vi "DEMO1.vi"() -> ()   [LabVIEW 2018]
uses:
  <vilib>/Utility/miscctls.llb/LVPositionTypeDef.ctl
  RandomMoveBool.lvclass
  RandomMoveBool.lvclass/RandomMoveBool.ctl
panel:
  out "数值":i32
  in  "Color":u32(colorbox)=6618880
  in  "Stop":bool
  in  "Remove":bool
  in  "Add":bool
  out "10 9":bool caption="布尔6"
  out "5 9":bool caption="布尔5"
  out "3 9":bool caption="布尔4"
  out "4 9":bool caption="布尔5"
  out "6 9":bool caption="布尔3"
  out "9 9":bool caption="布尔4"
  out "7 9":bool caption="布尔6"
  out "2 9":bool caption="布尔5"
  out "1 9":bool caption="布尔4"
  out "8 9":bool caption="布尔7"
  out "10 10":bool caption="布尔6"
  out "5 10":bool caption="布尔5"
  out "3 10":bool caption="布尔4"
  out "4 10":bool caption="布尔5"
  out "6 10":bool caption="布尔3"
  out "9 10":bool caption="布尔4"
  out "7 10":bool caption="布尔6"
  out "2 10":bool caption="布尔5"
  out "1 10":bool caption="布尔4"
  out "8 10":bool caption="布尔7"
  out "10 5":bool caption="布尔6"
  out "5 5":bool caption="布尔5"
  out "3 5":bool caption="布尔4"
  out "4 5":bool caption="布尔5"
  out "6 5":bool caption="布尔3"
  out "9 5":bool caption="布尔4"
  out "7 5":bool caption="布尔6"
  out "2 5":bool caption="布尔5"
  out "1 5":bool caption="布尔4"
  out "8 5":bool caption="布尔7"
  out "10 6":bool caption="布尔6"
  out "5 6":bool caption="布尔5"
  out "3 6":bool caption="布尔4"
  out "4 6":bool caption="布尔5"
  out "6 6":bool caption="布尔3"
  out "9 6":bool caption="布尔4"
  out "7 6":bool caption="布尔6"
  out "2 6":bool caption="布尔5"
  out "1 6":bool caption="布尔4"
  out "8 6":bool caption="布尔7"
  out "10 7":bool caption="布尔6"
  out "5 7":bool caption="布尔5"
  out "3 7":bool caption="布尔4"
  out "4 7":bool caption="布尔5"
  out "6 7":bool caption="布尔3"
  out "9 7":bool caption="布尔4"
  out "7 7":bool caption="布尔6"
  out "2 7":bool caption="布尔5"
  out "1 7":bool caption="布尔4"
  out "8 7":bool caption="布尔7"
  out "10 8":bool caption="布尔6"
  out "5 8":bool caption="布尔5"
  out "3 8":bool caption="布尔4"
  out "4 8":bool caption="布尔5"
  out "6 8":bool caption="布尔3"
  out "9 8":bool caption="布尔4"
  out "7 8":bool caption="布尔6"
  out "2 8":bool caption="布尔5"
  out "1 8":bool caption="布尔4"
  out "8 8":bool caption="布尔7"
  out "10 3":bool caption="布尔6"
  out "5 3":bool caption="布尔5"
  out "3 3":bool caption="布尔4"
  out "4 3":bool caption="布尔5"
  out "6 3":bool caption="布尔3"
  out "9 3":bool caption="布尔4"
  out "7 3":bool caption="布尔6"
  out "2 3":bool caption="布尔5"
  out "1 3":bool caption="布尔4"
  out "8 3":bool caption="布尔7"
  out "10 4":bool caption="布尔6"
  out "5 4":bool caption="布尔5"
  out "3 4":bool caption="布尔4"
  out "4 4":bool caption="布尔5"
  out "6 4":bool caption="布尔3"
  out "9 4":bool caption="布尔4"
  out "7 4":bool caption="布尔6"
  out "2 4":bool caption="布尔5"
  out "1 4":bool caption="布尔4"
  out "8 4":bool caption="布尔7"
  out "10 2":bool caption="布尔6"
  out "5 2":bool caption="布尔5"
  out "3 2":bool caption="布尔4"
  out "4 2":bool caption="布尔5"
  out "6 2":bool caption="布尔3"
  out "9 2":bool caption="布尔4"
  out "7 2":bool caption="布尔6"
  out "2 2":bool caption="布尔5"
  out "1 2":bool caption="布尔4"
  out "8 2":bool caption="布尔7"
  out "10":bool caption="布尔6"
  out "5":bool caption="布尔5"
  out "3":bool caption="布尔4"
  out "4":bool caption="布尔5"
  out "6":bool caption="布尔3"
  out "9":bool caption="布尔4"
  out "7":bool caption="布尔6"
  out "2":bool caption="布尔5"
  out "1":bool caption="布尔4"
  out "8":bool caption="布尔7"
  out "数组":T1[](array[typedef])
  in  "frequency2":dbl=3.0 format="%#_13g"
  in  "frequency1":dbl=3.0 format="%#_13g"
  in  "?":enum16{"Random", "Sine", "Other"}(ring)
  in  "limit":dbl=150.0 format="%#_13g"
  in  "等待时间（毫秒）":u32 step=20
  in  "ChangeColor":bool
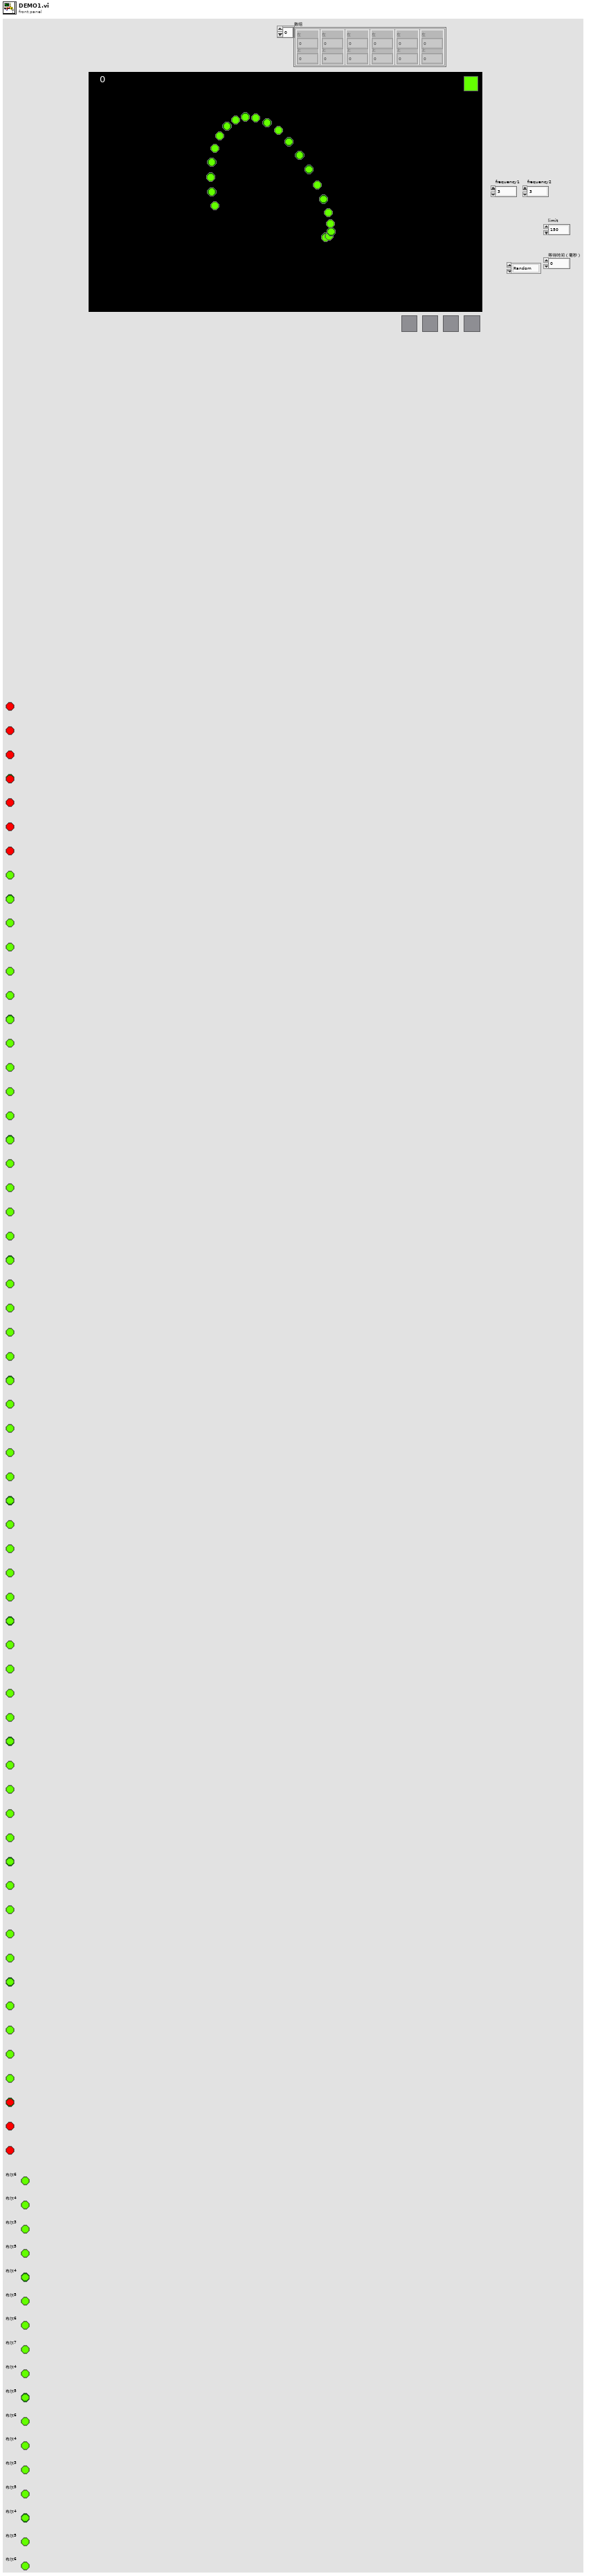
[diagram p1: front panel]
types:
  T1 = typedef "LVPositionTypeDef.ctl" = cluster{"Left":i32, "Top":i32}
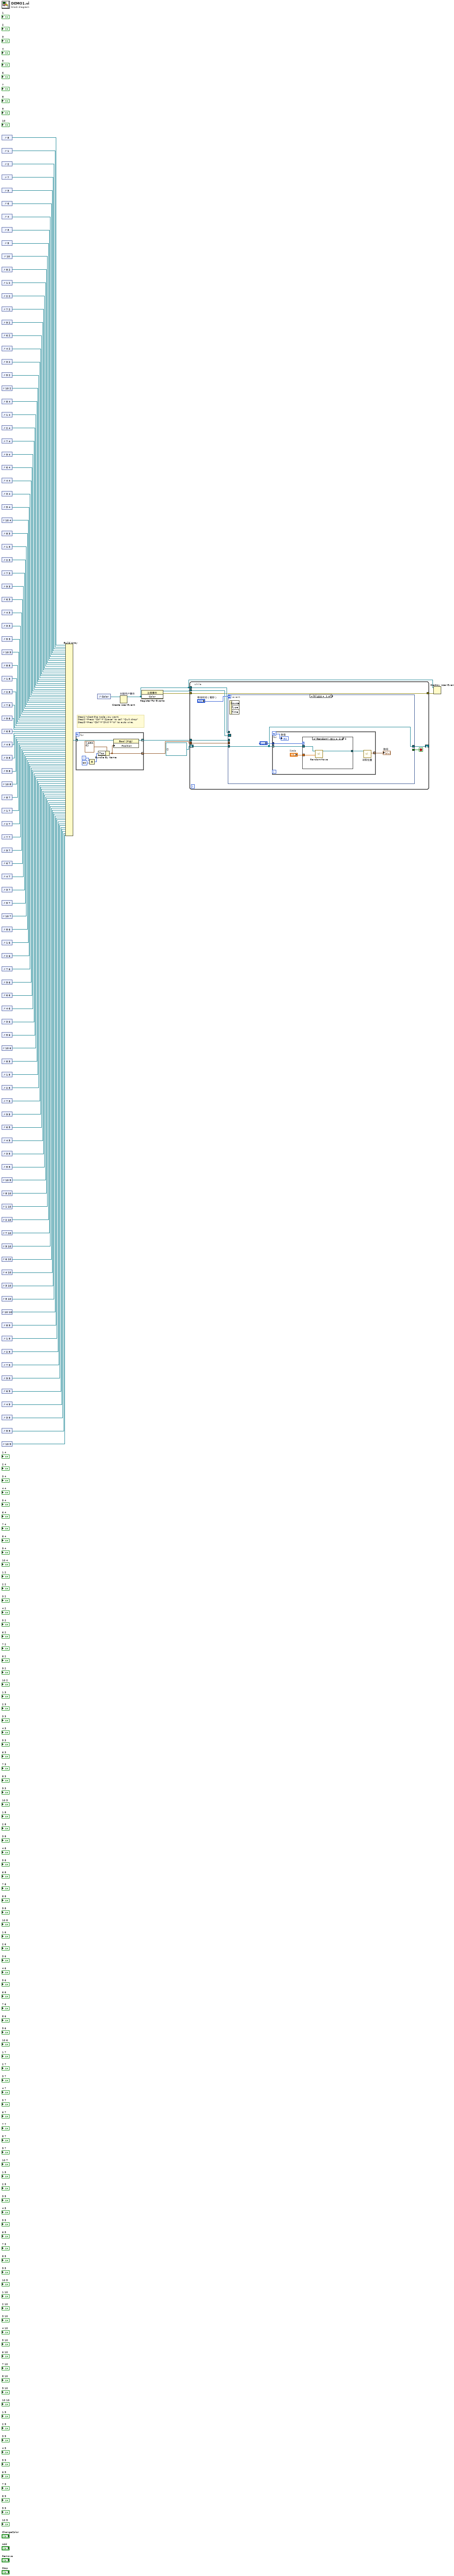
[diagram p0: block diagram]
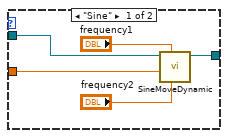
[diagram p2: hidden frame]
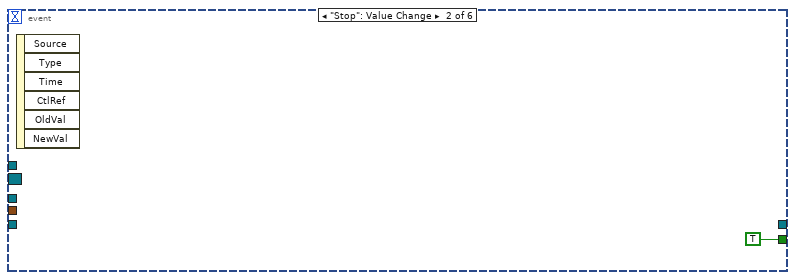
[diagram p3: hidden frame]
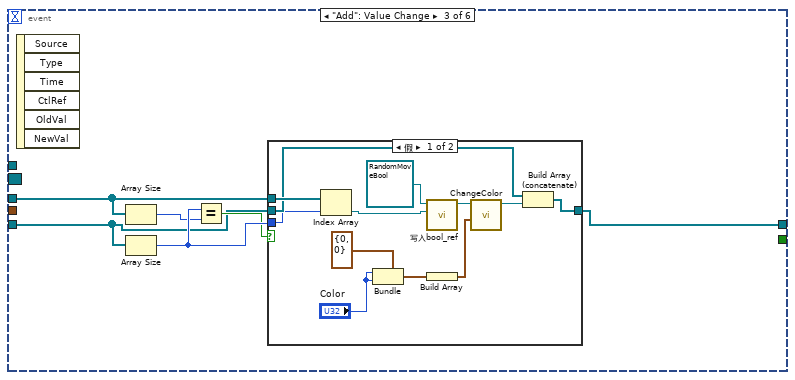
[diagram p4: hidden frame]
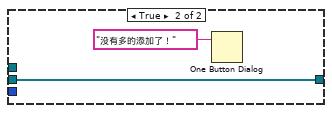
[diagram p5: hidden frame]
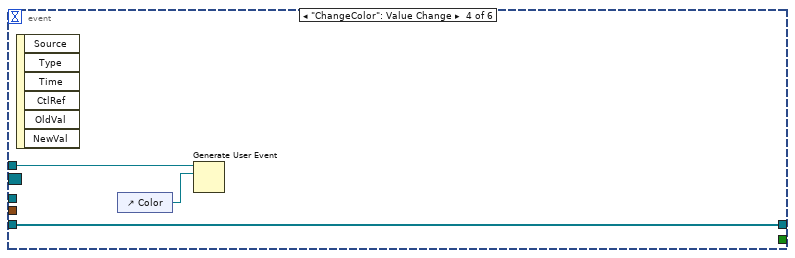
[diagram p6: hidden frame]
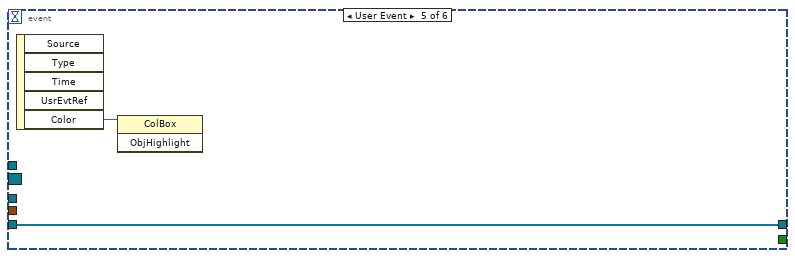
[diagram p7: hidden frame]
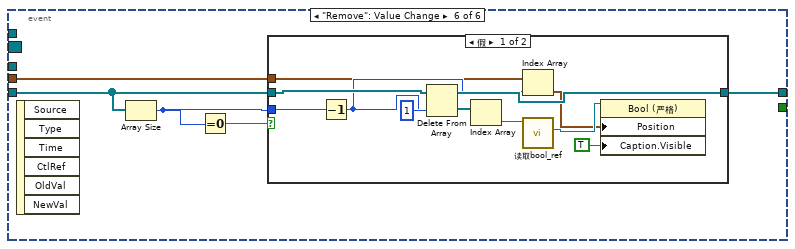
[diagram p8: hidden frame]
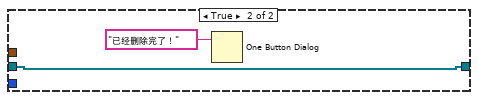
[diagram p9: hidden frame]
diagram:
  # "Step1>slect the node you want.\nStep2>Press \"Ctrl\"+\"Space\" to call \"Quik drop\"\nStep3>Pres \"Ctrl\"+\"Shit\"+\"W\" to auto wire."
  n1 = control-ref of="8"() -> (w101:refnum<vi>)
  n2 = control-ref of="1"() -> (w100:refnum<vi>)
  n3 = control-ref of="2"() -> (w99:refnum<vi>)
  n4 = control-ref of="7"() -> (w98:refnum<vi>)
  n5 = control-ref of="9"() -> (w97:refnum<vi>)
  n6 = control-ref of="6"() -> (w96:refnum<vi>)
  n7 = control-ref of="4"() -> (w95:refnum<vi>)
  n8 = control-ref of="3"() -> (w94:refnum<vi>)
  n9 = control-ref of="5"() -> (w93:refnum<vi>)
  n10 = control-ref of="10"() -> (w92:refnum<vi>)
  n11 = control-ref of="8 2"() -> (w91:refnum<vi>)
  n12 = control-ref of="1 2"() -> (w90:refnum<vi>)
  n13 = control-ref of="2 2"() -> (w89:refnum<vi>)
  n14 = control-ref of="7 2"() -> (w88:refnum<vi>)
  n15 = control-ref of="9 2"() -> (w87:refnum<vi>)
  n16 = control-ref of="6 2"() -> (w86:refnum<vi>)
  n17 = control-ref of="4 2"() -> (w85:refnum<vi>)
  n18 = control-ref of="3 2"() -> (w84:refnum<vi>)
  n19 = control-ref of="5 2"() -> (w83:refnum<vi>)
  n20 = control-ref of="10 2"() -> (w82:refnum<vi>)
  n21 = control-ref of="8 4"() -> (w81:refnum<vi>)
  n22 = control-ref of="1 4"() -> (w80:refnum<vi>)
  n23 = control-ref of="2 4"() -> (w79:refnum<vi>)
  n24 = control-ref of="7 4"() -> (w78:refnum<vi>)
  n25 = control-ref of="9 4"() -> (w77:refnum<vi>)
  n26 = control-ref of="6 4"() -> (w76:refnum<vi>)
  n27 = control-ref of="4 4"() -> (w75:refnum<vi>)
  n28 = control-ref of="3 4"() -> (w74:refnum<vi>)
  n29 = control-ref of="5 4"() -> (w73:refnum<vi>)
  n30 = control-ref of="10 4"() -> (w72:refnum<vi>)
  n31 = control-ref of="8 3"() -> (w71:refnum<vi>)
  n32 = control-ref of="1 3"() -> (w70:refnum<vi>)
  n33 = control-ref of="2 3"() -> (w69:refnum<vi>)
  n34 = control-ref of="7 3"() -> (w68:refnum<vi>)
  n35 = control-ref of="9 3"() -> (w67:refnum<vi>)
  n36 = control-ref of="6 3"() -> (w66:refnum<vi>)
  n37 = control-ref of="4 3"() -> (w65:refnum<vi>)
  n38 = control-ref of="3 3"() -> (w64:refnum<vi>)
  n39 = control-ref of="5 3"() -> (w63:refnum<vi>)
  n40 = control-ref of="10 3"() -> (w62:refnum<vi>)
  n41 = control-ref of="8 8"() -> (w61:refnum<vi>)
  n42 = control-ref of="1 8"() -> (w60:refnum<vi>)
  n43 = control-ref of="2 8"() -> (w59:refnum<vi>)
  n44 = control-ref of="7 8"() -> (w58:refnum<vi>)
  n45 = control-ref of="9 8"() -> (w57:refnum<vi>)
  n46 = control-ref of="6 8"() -> (w56:refnum<vi>)
  n47 = control-ref of="4 8"() -> (w55:refnum<vi>)
  n48 = control-ref of="3 8"() -> (w54:refnum<vi>)
  n49 = control-ref of="5 8"() -> (w53:refnum<vi>)
  n50 = control-ref of="10 8"() -> (w52:refnum<vi>)
  n51 = control-ref of="8 7"() -> (w51:refnum<vi>)
  n52 = control-ref of="1 7"() -> (w50:refnum<vi>)
  n53 = control-ref of="2 7"() -> (w49:refnum<vi>)
  n54 = control-ref of="7 7"() -> (w48:refnum<vi>)
  n55 = control-ref of="9 7"() -> (w47:refnum<vi>)
  n56 = control-ref of="6 7"() -> (w46:refnum<vi>)
  n57 = control-ref of="4 7"() -> (w45:refnum<vi>)
  n58 = control-ref of="3 7"() -> (w44:refnum<vi>)
  n59 = control-ref of="5 7"() -> (w43:refnum<vi>)
  n60 = control-ref of="10 7"() -> (w42:refnum<vi>)
  n61 = control-ref of="8 6"() -> (w41:refnum<vi>)
  n62 = control-ref of="1 6"() -> (w40:refnum<vi>)
  n63 = control-ref of="2 6"() -> (w39:refnum<vi>)
  n64 = control-ref of="7 6"() -> (w38:refnum<vi>)
  n65 = control-ref of="9 6"() -> (w37:refnum<vi>)
  n66 = control-ref of="6 6"() -> (w36:refnum<vi>)
  n67 = control-ref of="4 6"() -> (w35:refnum<vi>)
  n68 = control-ref of="3 6"() -> (w34:refnum<vi>)
  n69 = control-ref of="5 6"() -> (w33:refnum<vi>)
  n70 = control-ref of="10 6"() -> (w32:refnum<vi>)
  n71 = control-ref of="8 5"() -> (w31:refnum<vi>)
  n72 = control-ref of="1 5"() -> (w30:refnum<vi>)
  n73 = control-ref of="2 5"() -> (w29:refnum<vi>)
  n74 = control-ref of="7 5"() -> (w28:refnum<vi>)
  n75 = control-ref of="9 5"() -> (w27:refnum<vi>)
  n76 = control-ref of="6 5"() -> (w26:refnum<vi>)
  n77 = control-ref of="4 5"() -> (w25:refnum<vi>)
  n78 = control-ref of="3 5"() -> (w24:refnum<vi>)
  n79 = control-ref of="5 5"() -> (w23:refnum<vi>)
  n80 = control-ref of="10 5"() -> (w22:refnum<vi>)
  n81 = control-ref of="8 10"() -> (w21:refnum<vi>)
  n82 = control-ref of="1 10"() -> (w20:refnum<vi>)
  n83 = control-ref of="2 10"() -> (w19:refnum<vi>)
  n84 = control-ref of="7 10"() -> (w18:refnum<vi>)
  n85 = control-ref of="9 10"() -> (w17:refnum<vi>)
  n86 = control-ref of="6 10"() -> (w16:refnum<vi>)
  n87 = control-ref of="4 10"() -> (w15:refnum<vi>)
  n88 = control-ref of="3 10"() -> (w14:refnum<vi>)
  n89 = control-ref of="5 10"() -> (w13:refnum<vi>)
  n90 = control-ref of="10 10"() -> (w12:refnum<vi>)
  n91 = control-ref of="8 9"() -> (w11:refnum<vi>)
  n92 = control-ref of="1 9"() -> (w10:refnum<vi>)
  n93 = control-ref of="2 9"() -> (w9:refnum<vi>)
  n94 = control-ref of="7 9"() -> (w8:refnum<vi>)
  n95 = control-ref of="9 9"() -> (w7:refnum<vi>)
  n96 = control-ref of="6 9"() -> (w6:refnum<vi>)
  n97 = control-ref of="4 9"() -> (w5:refnum<vi>)
  n98 = control-ref of="3 9"() -> (w4:refnum<vi>)
  n99 = control-ref of="5 9"() -> (w3:refnum<vi>)
  n100 = control-ref of="10 9"() -> (w2:refnum<vi>)
  n101 = Build Array(w101, w100, w99, w98, w97, w96, w95, w94, w93, w92, w91, w90, w89, w88, w87, w86, w85, w84, w83, w82, w81, w80, w79, w78, w77, w76, w75, w74, w73, w72, w71, w70, w69, w68, w67, w66, w65, w64, w63, w62, w61, w60, w59, w58, w57, w56, w55, w54, w53, w52, w51, w50, w49, w48, w47, w46, w45, w44, w43, w42, w41, w40, w39, w38, w37, w36, w35, w34, w33, w32, w31, w30, w29, w28, w27, w26, w25, w24, w23, w22, w21, w20, w19, w18, w17, w16, w15, w14, w13, w12, w11, w10, w9, w8, w7, w6, w5, w4, w3, w2) -> (w1:refnum<vi>[])
  n102 = for {
    tunnel: w1 -> [w116] mode=indexing
    tunnel: [w111] -> w108 mode=indexing
    tunnel: [w110] -> w107 mode=indexing
    i -> [w114]
    n103 = Multiply(x=w114, y=60) -> (x*y=w113:i32)
    n104 = Bundle By Name(cluster=T1 {"Left"=-650, "Top"=0} ("位置"), "Top"=w113) -> (w110:T1)
    n105 = property class="Bool (严格)"(reference=w116, "Position"=w110) -> (reference out=w111:refnum<vi>)  [unwired: 1 in, 1 out]
  }
  n106 = control-ref of="Color"() -> (w106:refnum<vi>)
  n107 = Create User Event "创建用户事件"(user event datatype=w106) -> (user event=w104:refnum<user-event>)  [unwired: 1 in, 1 out]
  n108 = register-events(w104) -> (reference out=w105:refnum<event-registration>, error out=w102:errorcluster)  [unwired: 2 in]
  n109 = while {
    shift-right: [w123] -> _
    shift-left: refnum<class "RandomMoveBool.lvclass">[] [] -> [w124]
    tunnel: w108 -> [w122]
    tunnel: w107 -> [w120]
    tunnel: w105 -> [w119]
    tunnel: w104 -> [w118]
    tunnel: [w117] -> w103
    tunnel: w102 -> [w117]
    stop <- w125 stop-if-true
    n110 = event shown="[0] 超时" {
      selector: w119 -> [_ _ _ _ _ _]
      dyn-events: _ -> [_ _ _ _ _ _]
      timeout: "等待时间（毫秒）" -> [_ _ _ _ _ _]
      tunnel: [_ TRUE _ _ _ _] -> w125
      tunnel: w124 -> [w128 _ w145 w166 w167 w172]
      tunnel: [w128 _ w144 w166 w167 w171] -> w123
      tunnel: w122 -> [_ _ w149 _ _ _]
      tunnel: w120 -> [_ _ _ _ _ w169]
      tunnel: w118 -> [_ _ _ w165 _ _]
      event Timeout {
        n111 = event-data() -> ()  [unwired: 1 in, 3 out]
        n112 = for {
          N -> [w129]
          tunnel: w128 -> [w133] mode=indexing
          tunnel: "?" -> [w132]
          tunnel: [w130] -> w126 mode=indexing
          n113 = case shown="\"Random\", 默认" w132 {
            tunnel: "limit" -> [w138 w142]
            tunnel: w133 -> [w139 w141]
            tunnel: [w135 w140] -> w131
            frame "Sine" {
              n114 = call-dynamic "SineMoveDynamic.vi"("frequency2"="frequency2", "frequency1"="frequency1", "limit"=w138, "RandomMoveBool 输入"=w139) -> ("RandomMoveBool 输出"=w135:refnum<class "RandomMoveBool.lvclass">)  [unwired: 6 in, 1 out]
            }
            frame "Random", Default {
              n115 = call "RandomMove.vi"("limit"=w142, "RandomMoveBool 输入"=w141) -> ("RandomMoveBool 输出"=w140:refnum<class "RandomMoveBool.lvclass">)  [unwired: 8 in, 1 out]
            }
          }
          n116 = call "读取位置.vi"("RandomMoveBool输入"=w131) -> ("Position"=w130:T1)  [unwired: 8 in, 2 out]
          "数值" <- w129
        }
        "数组" <- w126
      }
      event "Stop": Value Change {
        n117 = event-data() -> ()  [unwired: 1 in, 6 out]
      }
      event "Add": Value Change {
        n118 = event-data() -> ()  [unwired: 1 in, 6 out]
        n119 = Array Size(array=w149) -> (size(s)=w147:i32)
        n120 = Array Size(array=w145) -> (size(s)=w148:i32)
        n121 = Equal?(x=w148, y=w147) -> (x = y?=w146:bool)
        n122 = case shown="假" w146 {
          tunnel: w149 -> [w159 _]
          tunnel: w148 -> [w156 _]
          tunnel: w145 -> [w158 w163]
          tunnel: [w157 w163] -> w144
          frame False {
            n123 = Index Array(array=w159, index=w156) -> (element=w160:refnum<vi>)
            n124 = Bundle(cluster=cluster{u32, u32} {0, 0}, "Color", "Color") -> (w154:cluster{u32, u32})
            n125 = call "写入bool_ref.vi"("布尔8 5"=w160, "RandomMoveBool输入"=refnum<class "RandomMoveBool.lvclass"> refnum ("RandomMoveBool.lvclass")) -> ("RandomMoveBool输出"=w151:refnum<class "RandomMoveBool.lvclass">)  [unwired: 8 in, 1 out]
            n126 = Build Array(w154) -> (w155:cluster{u32, u32}[])
            n127 = call-dynamic "ChangeColor.vi"("颜色[4]"=w155, "RandomMoveBool 输入"=w151) -> ("RandomMoveBool 输出"=w150:refnum<class "RandomMoveBool.lvclass">)  [unwired: 8 in, 1 out]
            n128 = Build Array (concatenate)(w158, w150) -> (w157:refnum<class "RandomMoveBool.lvclass">[])
          }
          frame True {
            n129 = One Button Dialog(message="没有多的添加了！" ("消息")) -> ()  [unwired: 1 in, 1 out]
          }
        }
      }
      event "ChangeColor": Value Change {
        n130 = event-data() -> ()  [unwired: 1 in, 6 out]
        n131 = control-ref of="Color"() -> (w164:refnum<vi>)
        n132 = Generate User Event(user event=w165, event data cluster=w164) -> ()  [unwired: 2 in, 2 out]
      }
      event User Event {
        n133 = event-data() -> ("Color"=w168:refnum<vi>)  [unwired: 1 in, 4 out]
        n134 = invoke class="ColBox" method="ObjHighlight"(reference=w168) -> ()  [unwired: 2 in, 3 out]
      }
      event "Remove": Value Change {
        n135 = event-data() -> ()  [unwired: 1 in, 6 out]
        n136 = Array Size(array=w172) -> (size(s)=w170:i32)
        n137 = Equal To 0?(x=w170) -> (x = 0?=w173:bool)
        n138 = case shown="假" w173 {
          tunnel: w172 -> [w184 w185]
          tunnel: [w183 w185] -> w171
          tunnel: w170 -> [w181 _]
          tunnel: w169 -> [w176 _]
          frame False {
            n139 = Decrement(x=w181) -> (x-1=w177:i32)
            n140 = Delete From Array(array=w184, length=1 ("长度"), index=w177) -> (deleted portion=w180:refnum<class "RandomMoveBool.lvclass">[], array with subset deleted=w183:refnum<class "RandomMoveBool.lvclass">[])
            n141 = Index Array(array=w180) -> (element=w179:refnum<class "RandomMoveBool.lvclass">)  [unwired: 1 in]
            n142 = Index Array(array=w176, index=w177) -> (element=w175:T1)
            n143 = call "读取bool_ref.vi"("RandomMoveBool输入"=w179) -> ("bool_ref"=w178:refnum<vi>)  [unwired: 8 in, 2 out]
            n144 = property class="Bool (严格)"(reference=w178, "Position"=w175, "Caption.Visible"=TRUE ("标题.可见")) -> ()  [unwired: 1 in, 2 out]
          }
          frame True {
            n145 = One Button Dialog(message="已经删除完了！" ("消息")) -> ()  [unwired: 1 in, 1 out]
          }
        }
      }
    }
  }
  n146 = Destroy User Event(user event=w104, error in=w103) -> ()  [unwired: 1 out]
